vi "Add to Tree.vi"(5 "Child Position":i32, 6 "Display Text Override":string, 7 "Add children? (T)":bool=TRUE, 8 "error in (no error)":errorcluster, 9 "Parent Tag":string, 10 "Tree Manager in":refnum<class "Tree Manager.lvclass">, 11 "Element in":refnum<class "Element.lvclass">) -> (0 "error out":errorcluster, 2 "Tree Manager out":refnum<class "Tree Manager.lvclass">, 3 "Element out":refnum<class "Element.lvclass">)   [LabVIEW 2026, in "VILab.lvlib" / "Element.lvclass"]
uses:
  Element.lvclass
  Tree Manager/Tree Manager.lvclass
  Attribute/Attribute.lvclass
  Data Item/Data Item.lvclass
  Element.lvclass/Element.ctl
  C:/Users/acasalen/Documents/LabVIEW Data/Projects/VILab/source/SubVIs/Classes/Data Item/Data Item.lvclass
  C:/Users/acasalen/Documents/LabVIEW Data/Projects/VILab/source/SubVIs/Classes/Attribute/Attribute.lvclass
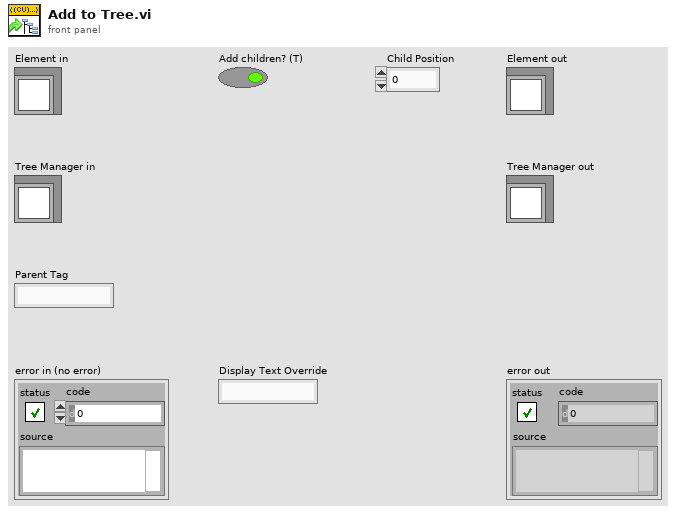
[diagram p1: front panel]
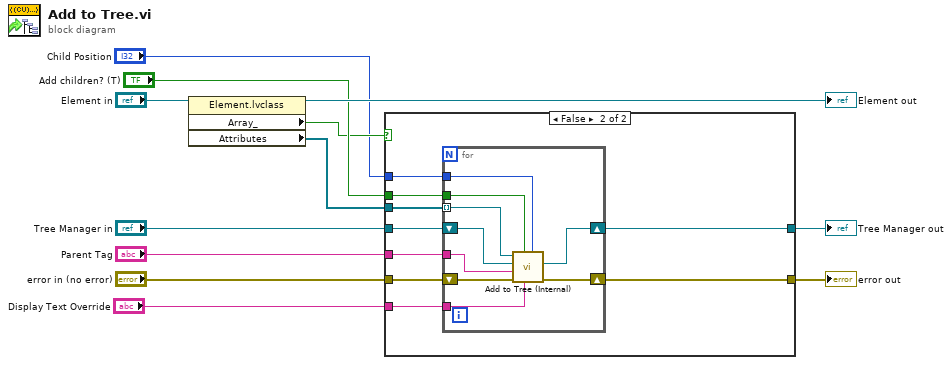
[diagram p0: block diagram]
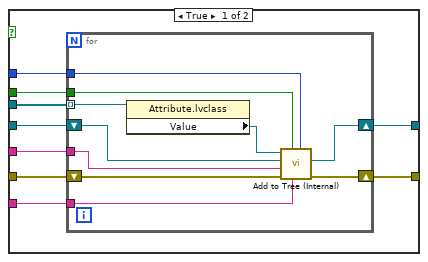
[diagram p2: hidden frame]
diagram:
  n1 = property class="Element.lvclass"(reference="Element in") -> (reference out=→"Element out":refnum<class "Element.lvclass">, "Array_"=w3:bool, "Attributes"=w4:refnum<class "Attribute.lvclass">[])  [unwired: 1 in, 1 out]
  n2 = case shown="False" w3 {
    tunnel: "error in (no error)" -> [w21 w40]
    tunnel: "Parent Tag" -> [w20 w39]
    tunnel: "Tree Manager in" -> [w19 w38]
    tunnel: [w18 w37] -> w7
    tunnel: [w17 w36] -> w6
    tunnel: "Add children? (T)" -> [w16 w35]
    tunnel: w4 -> [w15 w34]
    tunnel: "Child Position" -> [w14 w32]
    tunnel: "Display Text Override" -> [w13 w33]
    frame True {
      n3 = for {
        tunnel: w15 -> [w25] mode=indexing
        tunnel: w20 -> [w30]
        shift-right: [w27] -> w17
        shift-left: w21 -> [w31]
        shift-right: [w28] -> w18
        shift-left: w19 -> [w29]
        tunnel: w16 -> [w26]
        tunnel: w14 -> [w23]
        tunnel: w13 -> [w22]
        n4 = property class="Attribute.lvclass"(reference=w25) -> ("Value"=w24:refnum<class "Data Item.lvclass">)  [unwired: 1 in, 2 out]
        n5 = call "Add to Tree (Internal).vi"("Child Position"=w23, "Display Text Override"=w22, "Add children? (F)"=w26, "error in (no error)"=w31, "Parent Tag"=w30, "Tree Manager in"=w29, "Data Item in"=w24) -> ("error out"=w27:errorcluster, "Tree Manager out"=w28:refnum<class "Tree Manager.lvclass">)  [unwired: 1 in, 2 out]
      }
    }
    frame False {
      n6 = for {
        tunnel: w34 -> [w49] mode=indexing
        tunnel: w39 -> [w47]
        shift-right: [w44] -> w36
        shift-left: w40 -> [w48]
        shift-right: [w45] -> w37
        shift-left: w38 -> [w46]
        tunnel: w35 -> [w43]
        tunnel: w33 -> [w42]
        tunnel: w32 -> [w41]
        n7 = call "Add to Tree (Internal).vi"("Child Position"=w41, "Display Text Override"=w42, "Add children? (F)"=w43, "error in (no error)"=w48, "Parent Tag"=w47, "Tree Manager in"=w46, "Data Item in"=w49) -> ("error out"=w44:errorcluster, "Tree Manager out"=w45:refnum<class "Tree Manager.lvclass">)  [unwired: 1 in, 2 out]
      }
    }
  }
  "error out" <- w6
  "Tree Manager out" <- w7
